vi "Turn On.vi"(0 "Interface_object in":refnum<class "SwitchableDevice.lvclass">, 5 "error in (no error)":errorcluster) -> (14 "Interface_object out":refnum<class "SwitchableDevice.lvclass">, 19 "error out":errorcluster)   [LabVIEW 2018, in "SwitchableDevice.lvclass"]
doc: "AZ Interface method template"
uses:
  SwitchableDevice.lvclass
  SwitchableDevice.lvclass/SwitchableDevice.ctl
panel:
  # "Add terminals, connect them to terminal pattern,\nand save the method.\n\nDo not edit BD of this method"
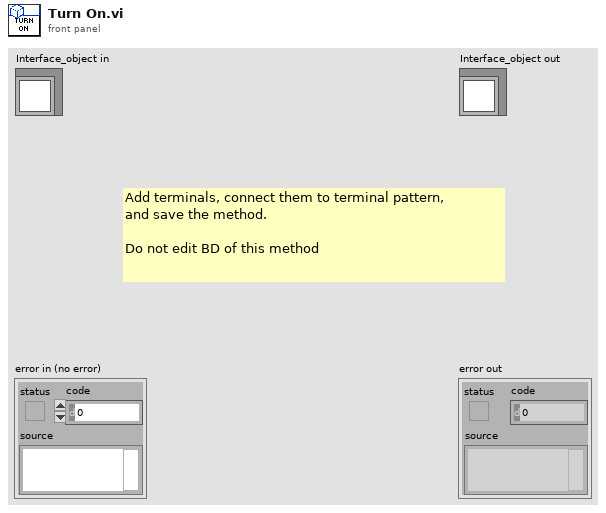
[diagram p1: front panel]
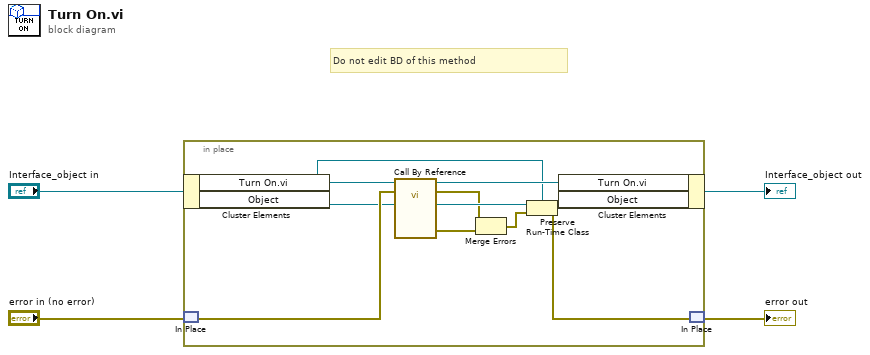
[diagram p0: block diagram]
diagram:
  # "Do not edit BD of this method"
  n1 = in-place {
    n2 = in-place-cluster #1("Interface_object in") -> ("Turn On.vi"=w14:refnum<vi>, "Object"=w7:refnum<class>)
    n3 = in-place-match #2("error in (no error)") -> (w11:errorcluster)
    n4 = call-by-ref "?"(reference=w14, error in=w11, "AZ_Interface in"=w7) -> (reference out=w13:refnum<vi>, error out=w9:errorcluster, "AZ_Interface out"=w12:refnum<class>, 19:"error out"=w10:errorcluster)  [unwired: 17 in]
    n5 = Merge Errors(w9, w10) -> (w6:errorcluster)
    n6 = Preserve Run-Time Class(object in=w12, error in=w6, 2:w7) -> (object out=w8:refnum<class>, error out=w5:errorcluster)
    n7 = in-place-cluster #1("Turn On.vi"=w13, "Object"=w8) -> (→"Interface_object out":refnum<class "SwitchableDevice.lvclass">)
    n8 = in-place-match #2(w5) -> (→"error out":errorcluster)
  }
